vi "Batt_DataLog.vi"(0 "Start 2":bool=TRUE) -> (1 "error out":errorcluster)   [LabVIEW 2016]
uses:
  MGCC_DataLog_global.vi
  Global tdms reference.vi
  Communication/Global communication.vi
  <vilib>/Utility/error.llb/Error Cluster From Error Code.vi
  Finite State Machine (He Yin)/Sub-VIs/MGCC_FntStaMach_gobal.vi
  Abnormal Fault State Control (He Yin)/Sub_VIs/Fault_Abnormal_state.vi
  <vilib>/ErrorRing/Error Ring.xnode
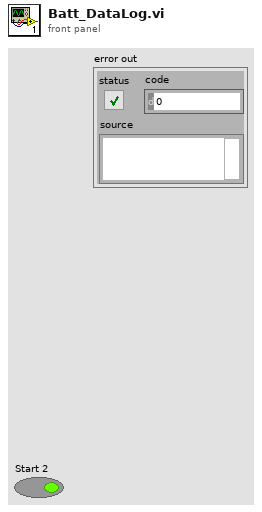
[diagram p1: front panel]
types:
  T1 = enum16{"open", "open or create", "create or replace", "create", "open (read-only)"}
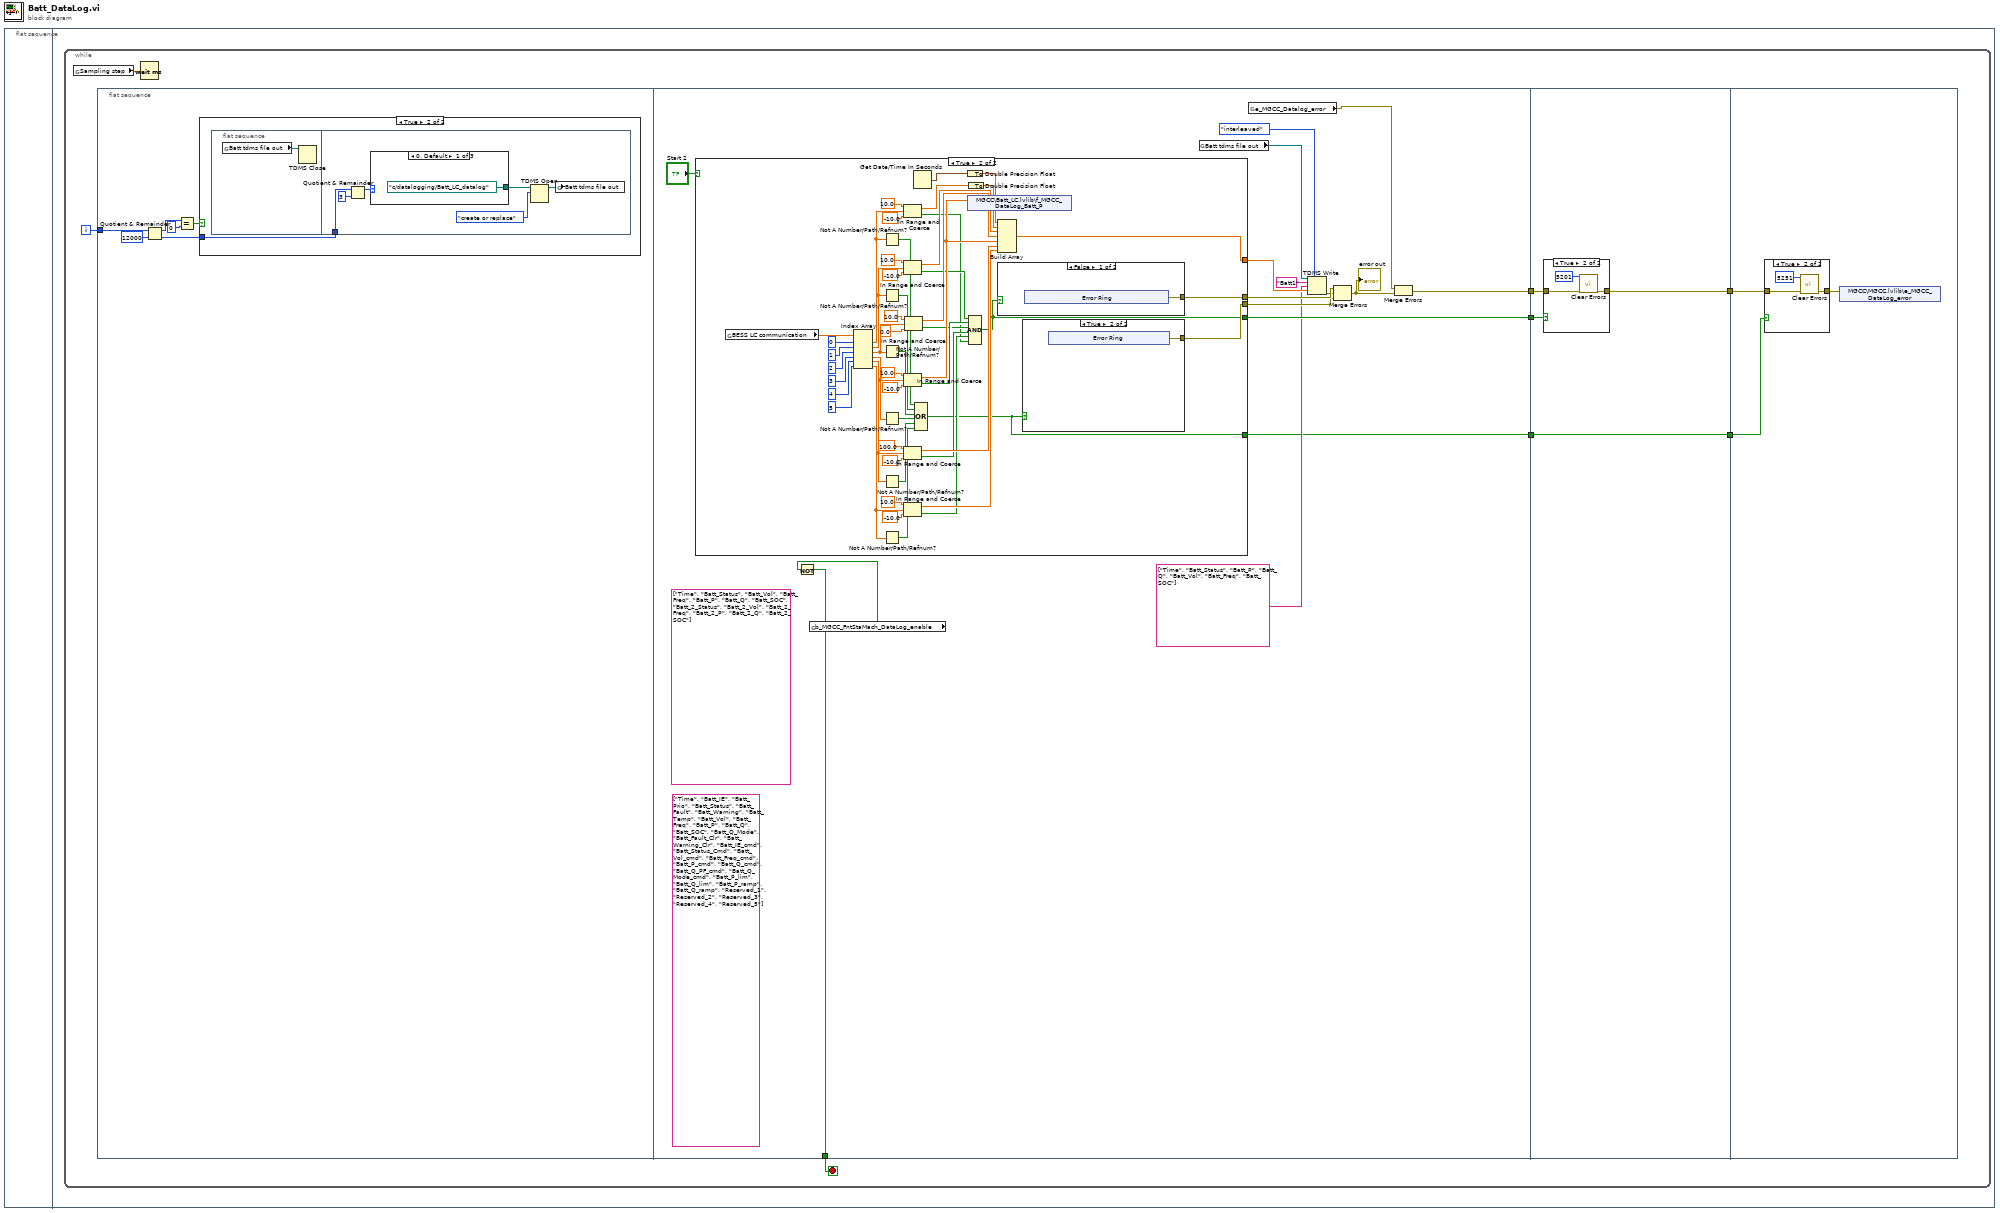
[diagram p0: block diagram]
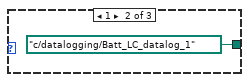
[diagram p3: hidden frame]
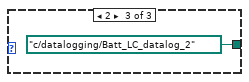
[diagram p4: hidden frame]
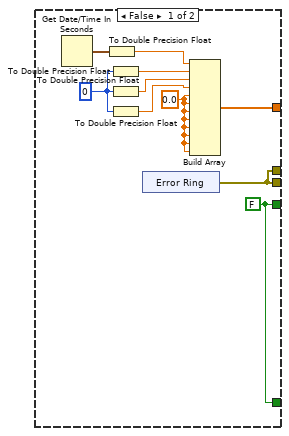
[diagram p5: hidden frame]
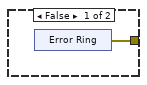
[diagram p6: hidden frame]
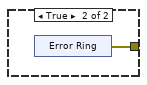
[diagram p7: hidden frame]
diagram:
  n1 = flat-sequence {
    frame #0 {
    }
    frame #1 {
      n2 = while {
        i -> [w4]
        stop <- w8 stop-if-true
        n3 = global read "MGCC_DataLog_global.vi" "Sampling step"() -> (w5:dbl)
        n4 = flat-sequence {
          tunnel: w4 -> [w14]
          tunnel: [w37] -> w8
          tunnel: [w31] -> w7
          tunnel: [w30] -> w6
          tunnel: [w28] -> w1
          tunnel: w7 -> [w122]
          tunnel: w6 -> [w123]
          tunnel: [w121] -> w3
          tunnel: [w120] -> w2
          tunnel: w1 -> [w120]
          tunnel: w3 -> [w129]
          tunnel: w2 -> [w128]
          frame #0 {
            n5 = Quotient & Remainder(x=w14, y=12000) -> (x-y*floor(x/y)=w12:i32, floor(x/y)=w9:i32)
            n6 = Equal?(x=w12, y=0) -> (x = y?=w10:bool)
            n7 = case shown="True" w10 {
              tunnel: w9 -> [_ w15]
              frame False {
              }
              frame True {
                n8 = flat-sequence {
                  tunnel: w15 -> [w20]
                  frame #0 {
                    n9 = global read "Global tdms reference.vi" "Batt tdms file out"() -> (w16:refnum<k34>)
                    n10 = TDMS Close(11:w16) -> ()  [unwired: 1 in, 2 out]
                  }
                  frame #1 {
                    n11 = Quotient & Remainder(x=w20, y=3) -> (x-y*floor(x/y)=w18:i32)  [unwired: 1 out]
                    n12 = case shown="0, Default" w18 {
                      tunnel: [path "c:/datalogging/Batt_LC_datalog" ("file path (dialog if empty)") path "c:/datalogging/Batt_LC_datalog_1" ("file path (dialog if empty)") path "c:/datalogging/Batt_LC_datalog_2" ("file path (dialog if empty)")] -> w17
                      frame 0, Default {
                      }
                      frame 1 {
                      }
                      frame 2 {
                      }
                    }
                    n13 = TDMS Open(10:T1."create or replace" ("operation (0:open)"), 11:w17) -> (3:w22:refnum<k34>)  [unwired: 5 in, 1 out]
                    n14 = global write "Global tdms reference.vi" "Batt tdms file out"(w22) -> ()
                  }
                }
              }
            }
          }
          frame #1 {
            (unwired) string[] ["Time", "Batt_Status", "Batt_Vol", "Batt_Freq", "Batt_P", "Batt_Q", "Batt_SOC", "Batt_2_Status", "Batt_2_Vol", "Batt_2_Freq", "Batt_2_P", "Batt_2_Q", "Batt_2_SOC"] ("channel name(s) in (Untitled)")
            (unwired) string[] ["Time", "Batt_IE", "Batt_Prio", "Batt_Status", "Batt_Fault", "Batt_Warning", "Batt_Temp", "Batt_Vol", "Batt_Freq", "Batt_P", "Batt_Q", "Batt_SOC", "Batt_Q_Mode", "Batt_Fault_Clr", "Batt_Warning_Clr", "Batt_IE_cmd", "Batt_Status_Cmd", "Batt_Vol_cmd", "Batt_Freq_cmd", "Batt_P_cmd", "Batt_Q_cmd", "Batt_Q_PF_cmd", "Batt_Q_Mode_cmd", "Batt_P_lim", "Batt_Q_lim", "Batt_P_ramp", "Batt_Q_ramp", "Reserved_1", "Reserved_2", "Reserved_3", "Reserved_4", "Reserved_5"] ("channel name(s) in (Untitled)")
            n15 = case shown="True" "Start 2" {
              tunnel: [w45 w101] -> w39
              tunnel: [w43 w76] -> w36
              tunnel: [w43 w68] -> w33
              tunnel: [w42 w67] -> w30
              tunnel: [w42 w53] -> w28
              frame False {
                w42 = FALSE
                w50 = 0.0
                w46 = 0
                n16 = Get Date/Time In Seconds() -> (seconds since 1Jan1904=w44:timestamp)
                n17 = To Double Precision Float(number=w44) -> (double precision float=w47:dbl)
                n18 = To Double Precision Float(number=w46) -> (double precision float=w51:dbl)
                n19 = To Double Precision Float(number=w46) -> (double precision float=w49:dbl)
                n20 = To Double Precision Float(number=w46) -> (double precision float=w48:dbl)
                n21 = xnode "Error Ring"() -> ("error out"=w43:errorcluster)
                n22 = Build Array(w47, w51, w49, w48, w50, w50, w50, w50, w50, w50, w50, w50) -> (w45:dbl[])
              }
              frame True {
                n23 = global read "Global communication.vi" "BESS LC communication"() -> (w54:dbl[])
                n24 = Index Array(array=w54, index #1=0 ("index"), index #2=1 ("index"), index #3=2 ("index"), index #4=3 ("index"), index #5=4 ("index"), index #6=5 ("index")) -> (element #1=w65:dbl, element #2=w59:dbl, element #3=w58:dbl, element #4=w57:dbl, element #5=w56:dbl, element #6=w55:dbl)
                n25 = Not A Number/Path/Refnum?(number/path/refnum=w65) -> (NaN/Path/Refnum?=w74:bool)
                n26 = Not A Number/Path/Refnum?(number/path/refnum=w59) -> (NaN/Path/Refnum?=w73:bool)
                n27 = Not A Number/Path/Refnum?(number/path/refnum=w58) -> (NaN/Path/Refnum?=w72:bool)
                n28 = Not A Number/Path/Refnum?(number/path/refnum=w57) -> (NaN/Path/Refnum?=w71:bool)
                n29 = Not A Number/Path/Refnum?(number/path/refnum=w56) -> (NaN/Path/Refnum?=w70:bool)
                n30 = Not A Number/Path/Refnum?(number/path/refnum=w55) -> (NaN/Path/Refnum?=w69:bool)
                n31 = In Range and Coerce(upper limit=10.0, x=w65, lower limit=-10.0) -> (coerced(x)=w85:dbl, In Range?=w77:bool)
                n32 = In Range and Coerce(upper limit=10.0, x=w59, lower limit=-10.0) -> (coerced(x)=w99:dbl, In Range?=w82:bool)
                n33 = In Range and Coerce(upper limit=10.0, x=w57, lower limit=-10.0 ("x")) -> (coerced(x)=w96:dbl, In Range?=w81:bool)
                n34 = In Range and Coerce(upper limit=100.0, x=w56, lower limit=-10.0) -> (coerced(x)=w91:dbl, In Range?=w79:bool)
                n35 = In Range and Coerce(upper limit=10.0, x=w55, lower limit=-10.0) -> (coerced(x)=w88:dbl, In Range?=w78:bool)
                n36 = In Range and Coerce(upper limit=10.0, x=w58, lower limit=0.0) -> (coerced(x)=w94:dbl, In Range?=w80:bool)
                n37 = Get Date/Time In Seconds() -> (seconds since 1Jan1904=w100:timestamp)
                n38 = Compound Arithmetic op=OR(w74, w73, w72, w71, w70, w69) -> (w53:bool)
                n39 = To Double Precision Float(number=w100) -> (double precision float=w103:dbl)
                n40 = To Double Precision Float(number=w85) -> (double precision float=w102:dbl)
                n41 = shared-variable "MGCC\\Batt_LC.lvlib\\f_MGCC_DataLog_Batt_P"(w96) -> ()  [unwired: 1 in, 1 out]
                n42 = Compound Arithmetic op=AND(w82, w81, w80, w79, w78, w77) -> (w67:bool)
                n43 = Build Array(w103, w102, w99, w94, w96, w91, w88) -> (w101:dbl[])
                n44 = case shown="False" w67 {
                  tunnel: [w112 w118] -> w76
                  frame False {
                    n45 = xnode "Error Ring"() -> ("error out"=w112:errorcluster)
                  }
                  frame True {
                    n46 = xnode "Error Ring"() -> ("error out"=w118:errorcluster)
                  }
                }
                n47 = case shown="True" w53 {
                  tunnel: [w104 w106] -> w68
                  frame False {
                    n48 = xnode "Error Ring"() -> ("error out"=w104:errorcluster)
                  }
                  frame True {
                    n49 = xnode "Error Ring"() -> ("error out"=w106:errorcluster)
                  }
                }
              }
            }
            n50 = global read "MGCC_FntStaMach_gobal.vi" "b_MGCC_FntStaMach_DataLog_enable"() -> (w27:bool)
            n51 = Not(x=w27) -> (.not. x?=w37:bool)
            n52 = global read "Global tdms reference.vi" "Batt tdms file out"() -> (w32:refnum<k34>)
            n53 = global read "Fault_Abnormal_state.vi" "e_MGCC_Datalog_error"() -> (w26:errorcluster[])
            n54 = TDMS Write(0:w32, 1:enum16{"decimated", "interleaved"}."interleaved" ("data layout (0:decimated)"), 5:"Batt1" ("group name in (Untitled)"), 7:string[] ["Time", "Batt_Status", "Batt_P", "Batt_Q", "Batt_Vol", "Batt_Freq", "Batt_SOC"] ("channel name(s) in (Untitled)"), 9:w39) -> (15:w35:errorcluster)  [unwired: 1 in, 3 out]
            n55 = Merge Errors(w36, w35, w33) -> (w34:errorcluster)
            "error out" <- w34
            n56 = Merge Errors(w26, w34) -> (w31:errorcluster)
          }
          frame #2 {
            n57 = case shown="True" w123 {
              tunnel: w122 -> [w124 w127]
              tunnel: [w124 w125] -> w121
              frame False {
              }
              frame True {
                n58 = call <vilib>:"Clear Errors.vi"("error in (no error)"=w127, "specific error code to clear (0: all)"=5201) -> ("error out"=w125:errorcluster)  [unwired: 4 in, 1 out]
              }
            }
          }
          frame #3 {
            n59 = case shown="True" w128 {
              tunnel: w129 -> [w131 w134]
              tunnel: [w131 w132] -> w130
              frame False {
              }
              frame True {
                n60 = call <vilib>:"Clear Errors.vi"("error in (no error)"=w134, "specific error code to clear (0: all)"=5251) -> ("error out"=w132:errorcluster)  [unwired: 4 in, 1 out]
              }
            }
            n61 = shared-variable "MGCC\\MGCC.lvlib\\e_MGCC_DataLog_error"(w130) -> ()  [unwired: 1 in, 1 out]
          }
        }
        n62 = Wait (ms)(milliseconds to wait=w5) -> ()  [unwired: 1 out]
      }
    }
  }
